vi "phan_dieukhiengoc.vi"() -> ()   [LabVIEW 2019]
uses:
  <vilib>/Platform/TimedLoop/XDataNode/timing_clust.ctl
  <vilib>/Platform/TimedLoop/XDataNode/nitl_modes.ctl
  <vilib>/Platform/TimedLoop/XDataNode/wakeup.ctl
  <vilib>/platform/TimedLoop/XDataNode/XDataNode.xnode
  <vilib>/Platform/TimedLoop/XDataNode/XDNodeRunTimeDep.lvlib
  <vilib>/ptbypt/NI_PtbyPt.lvlib
panel:
  out "wdk":dbl
  out "phi_sp":dbl
  in  "Kiw":dbl
  in  "Kpw":dbl
  in  "Kdw":dbl=2.0
  out "phi_ph":dbl
  out "Vxdk":dbl
  out "Vydk":dbl
  in  "Kdv3":dbl
  in  "Kiv3":dbl=28.5
  in  "Kpv3":dbl=0.7
  in  "Kdv2":dbl
  in  "Kiv2":dbl=28.5
  in  "Kpv2":dbl=0.7
  out "Ts":dbl=10.0
  out "TOA DO 2":dbl[][](array[numeric])
  out "sailechxy":cluster{"e_phi":dbl, "e_x":dbl, "e_y":dbl}(graph)
  in  "Kdxy":dbl
  in  "Kixy":dbl
  in  "Kpxy":dbl=4.0
  in  "?":enum32{"DUONG 2", "DUONGTRON", "NHAP DIEM"}(tab)
  in  "xstart":dbl format="%#_13g"
  in  "xend":dbl=2.0
  in  "time2":dbl=10.0
  in  "R":dbl=0.8
  in  "phi_end":dbl=15.71
  in  "phi_start":dbl=3.14159 format="%#_13g"
  in  "time1":dbl=30.0
  out "output variable":dbl
  in  "y2":dbl
  in  "x1":dbl
  in  "x2":dbl
  in  "time3":dbl=10.0
  in  "x3":dbl
  in  "y3":dbl
  in  "y1":dbl
  in  "x4":dbl
  in  "y4":dbl
  out "V_ph":dbl
  out "w_ph3":dbl
  out "w_ph2":dbl
  out "w_ph1":dbl
  in  "RESETMAP":bool=TRUE caption="Reset"
  out "duty3":dbl
  out "duty2":dbl
  out "duty1":dbl
  in  "RESET":bool
  out "Y_sp":dbl
  out "X_sp":dbl
  out "Y_ph":dbl
  out "X_ph":dbl
  out "Map":cluster{"Y":dbl[], "Y":dbl[]}[](graph)
  out "V3_sp":dbl
  out "V3_ph":dbl
  out "VAN TOC":T1(graph)
  in  "Kdv1":dbl
  in  "Kiv1":dbl=28.5
  in  "Kpv1":dbl=0.7
  out "V2_ph":dbl
  out "V1_ph":dbl
  out "V2_sp":dbl
  out "V1_sp":dbl
  in  "START":bool
  # "HE THONG"
  # "PID VI TRI"
  # "PID TOC DO"
  # "DUTY"
  # "VI TRI DIEU KHIEN\n(m)"
  # "VI TRI PHAN HOI\n(m)"
  # "TOC DO PHAN HOI (rad/s)"
  # "VAN TOC DIEU KHIEN\n(m/s)"
  # "VAN TOC PHAN HOI\n(m/s)"
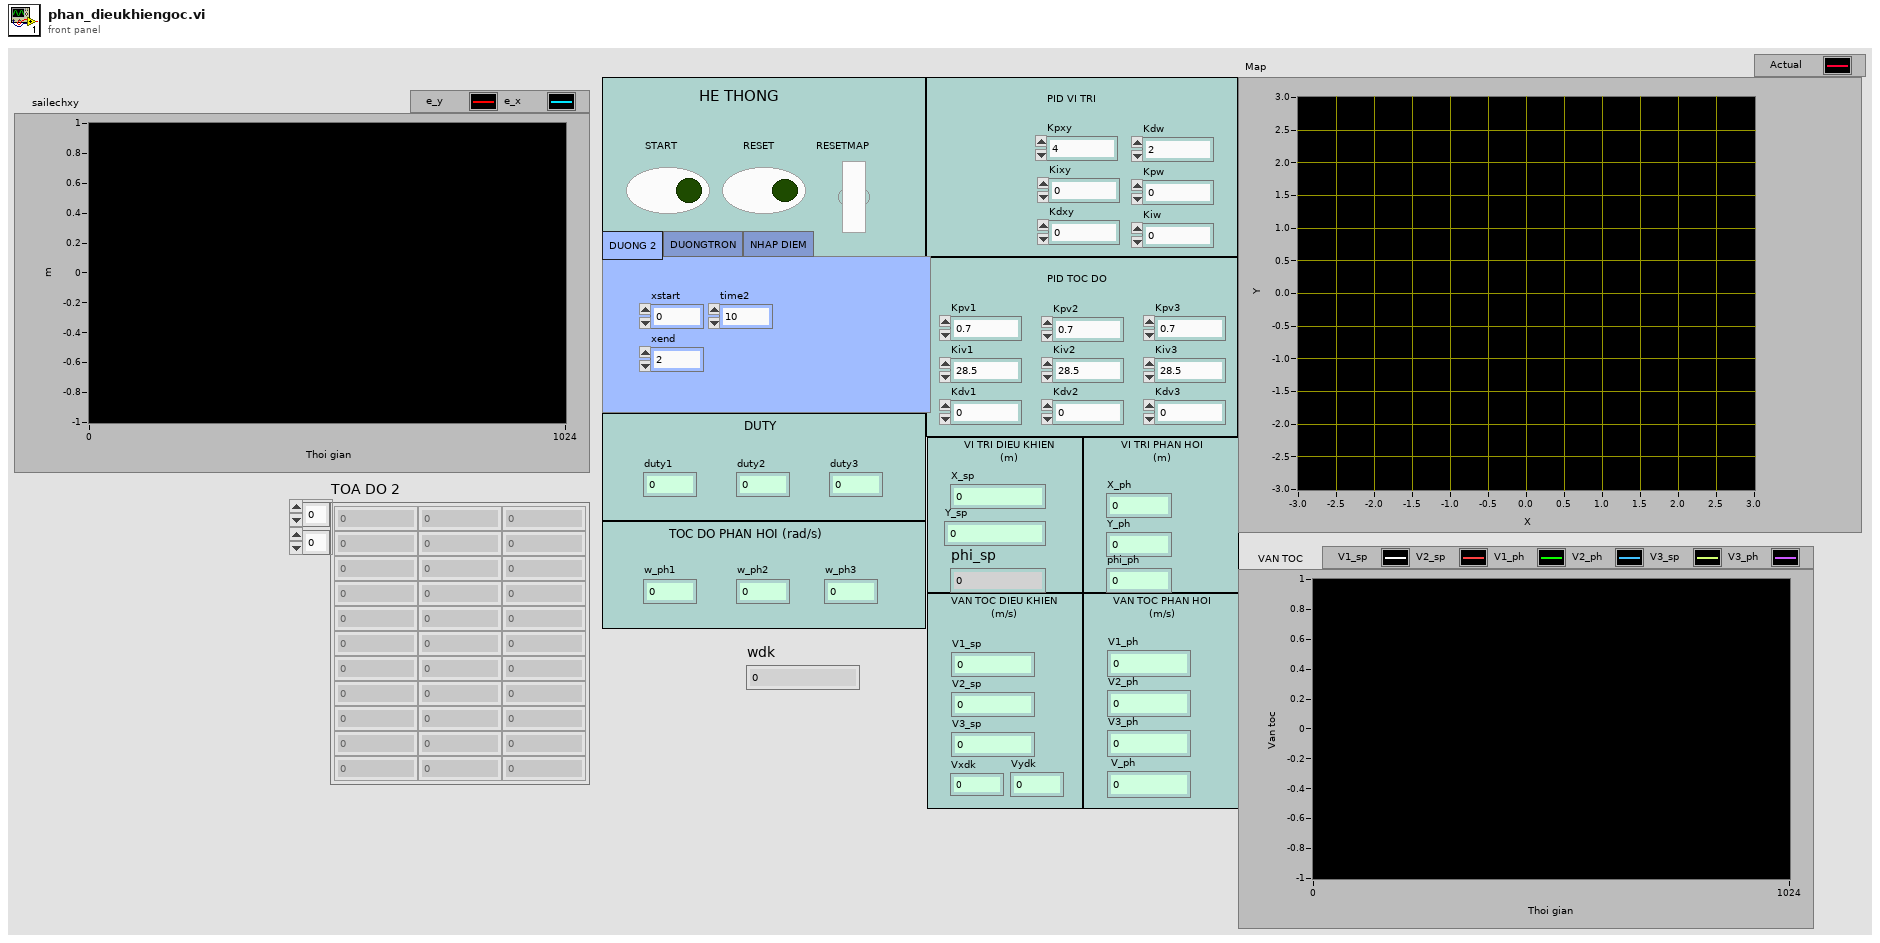
[diagram p1: front panel]
types:
  T1 = cluster{dbl, dbl, "V1_ph":dbl, "V2_ph":dbl, dbl, "V3_ph":dbl}
  T2 = typedef "XDNodeRunTimeDep.lvlib/timing_clust.ctl" = cluster{"Expected End [f-1]":u64, "Actual End [f-1]":u64, "Finished Late? [f-1]":bool, "Expected End [i-1]":u64, "Actual End [i-1]":u64, "Finished Late? [i-1]":bool, "Expected Start [i]":u64, "Actual Start [i]":u64, "Expected Start [f]":u64, "Actual Start [f]":u64, "Source Name":string, "Structure Name":string, "Period":i64, "Deadline":i64, "Offset":i64, "Start":i64, "Priority":i32, "Timeout":i32, "Mode":T3, "Wakeup Reason":T4, "Error":errorcluster, "Source Type":string, "Secondary Source Type":string, "Global End Time":u64, "Global Start Time":u64, "Frame Duration":u64, "Iteration Duration":u64, "Assigned CPU":i32, "I/O Scan Engine Mode":u32}
  T3 = typedef "XDNodeRunTimeDep.lvlib/nitl_modes.ctl" = enum32{"No Change", "Process missed periods, maintain original phase", "Discard missed periods, maintain original phase", "Process missed periods, ignore original phase", "Discard missed periods, ignore original phase"}
  T4 = typedef "XDNodeRunTimeDep.lvlib/wakeup.ctl" = enum32{"Normal", "Aborted", "Asynchronous wakeup", "Timing source error", "Timed loop error", "Timeout"}
  T5 = cluster{"V1_sp":dbl, "V_ph1":dbl, "V2_sp":dbl, "V_ph2":dbl, "V3_sp":dbl, "V_ph3":dbl}
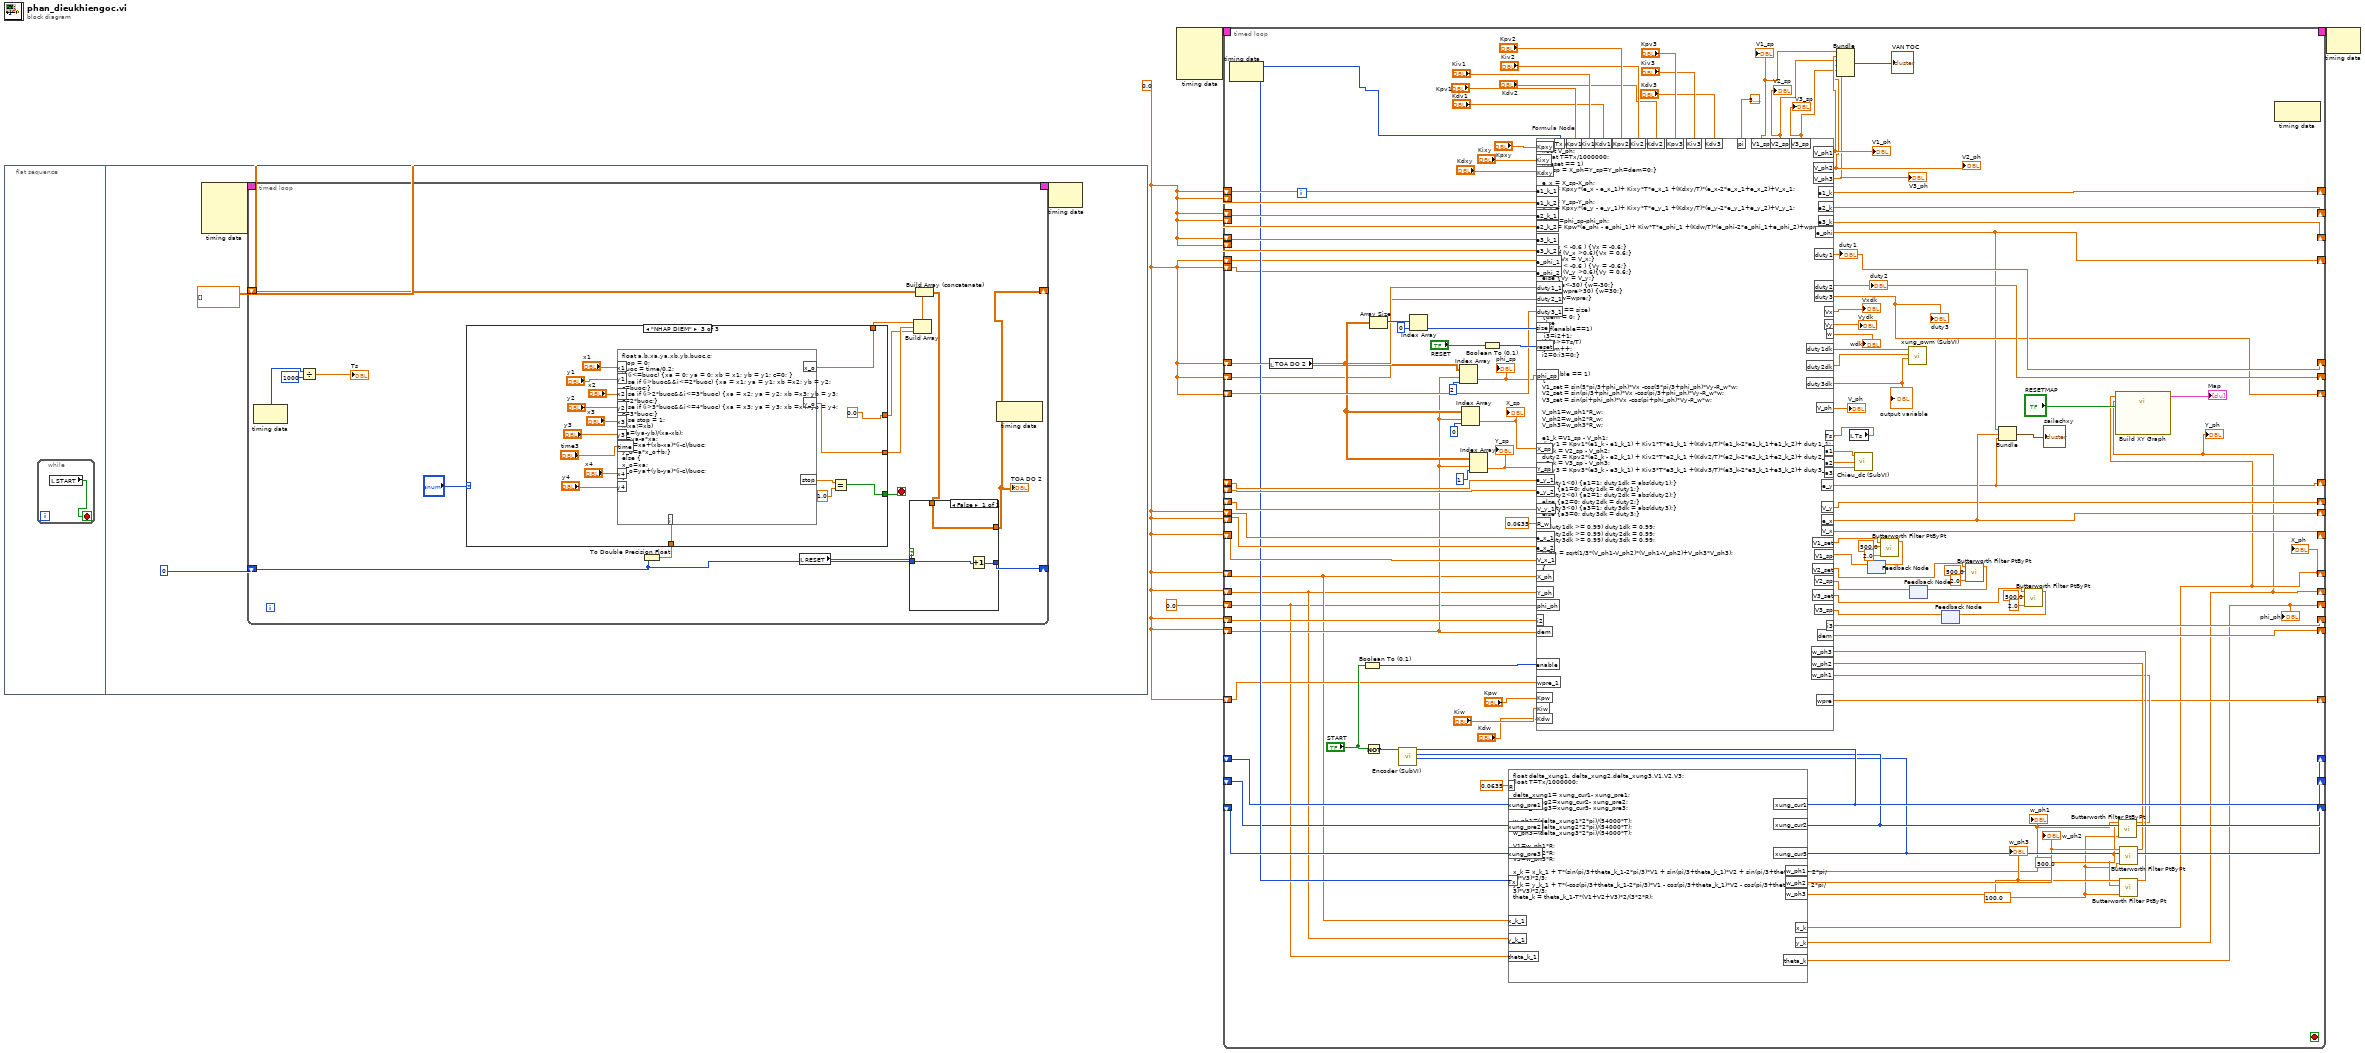
[diagram p0: block diagram]
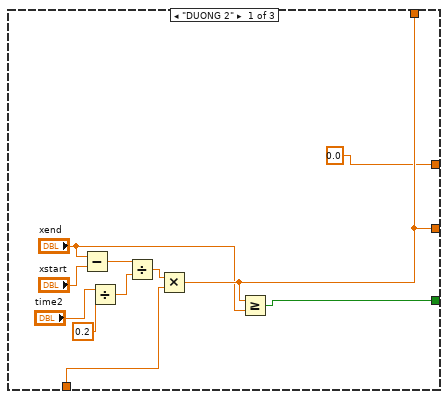
[diagram p2: hidden frame]
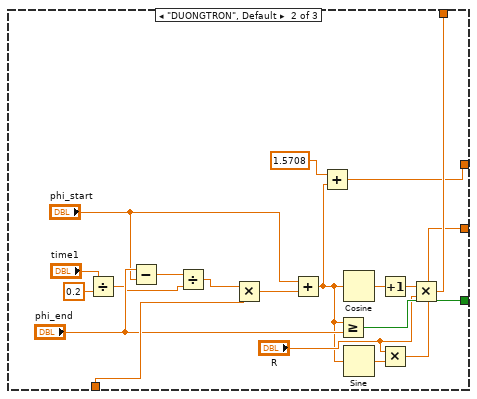
[diagram p3: hidden frame]
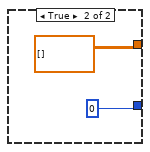
[diagram p4: hidden frame]
diagram:
  w2 = 0.0 ("e1")
  n1 = flat-sequence {
    frame #0 {
      n2 = while {
        stop <- w5 stop-if-true
        n3 = local read "START"() -> (w5:bool)
      }
    }
    frame #1 {
      n4 = node-c288() -> (w9:T2)  [unwired: 4 in]
      n5 = timed-loop {
        timing: w9 -> [_]
        timing-out: [_] -> w8
        shift-right: [w17] -> _
        shift-left: dbl[][] [] -> [w23]
        shift-right: [w21] -> _
        shift-left: 0 -> [w20]
        stop <- w14 stop-if-true
        n6 = node-c288() -> (w16:i64)  [unwired: 1 in]
        n7 = Divide(x=w16, y=i64 1000) -> (x/y=→"Ts":dbl)
        n8 = To Double Precision Float(number=w20) -> (double precision float=w25:dbl)
        n9 = case shown="\"NHAP DIEM\"" "?" {
          tunnel: w25 -> [w33 w55 w71]
          tunnel: [w32 w50 w64] -> w19
          tunnel: [w32 w49 w59] -> w18
          tunnel: [w30 w48 w61] -> w14
          tunnel: [0.0 w37 0.0] -> w10
          frame "DUONG 2" {
            n10 = Subtract(x="xend", y="xstart") -> (x-y=w35:dbl)
            n11 = Divide(x="time2", y=0.2) -> (x/y=w27:dbl)
            n12 = Divide(x=w35, y=w27) -> (x/y=w34:dbl)
            n13 = Multiply(x=w34, y=w33) -> (x*y=w32:dbl)
            n14 = Greater Or Equal?(x=w32, y="xend") -> (x >= y?=w30:bool)
          }
          frame "DUONGTRON", Default {
            n15 = Divide(x="time1", y=0.2) -> (x/y=w41:dbl)
            n16 = Subtract(x="phi_end", y="phi_start") -> (x-y=w45:dbl)
            n17 = Divide(x=w45, y=w41) -> (x/y=w44:dbl)
            n18 = Multiply(x=w44, y=w55) -> (x*y=w54:dbl)
            n19 = Add(x="phi_start", y=w54) -> (x+y=w38:dbl)
            n20 = Add(x=1.5708, y=w38) -> (x+y=w37:dbl)
            n21 = Greater Or Equal?(x=w38, y="phi_end") -> (x >= y?=w48:bool)
            n22 = Cosine(x=w38) -> (cos(x)=w53:dbl)
            n23 = Sine(x=w38) -> (sin(x)=w51:dbl)
            n24 = Increment(x=w53) -> (x+1=w52:dbl)
            n25 = Multiply(x="R", y=w51) -> (x*y=w49:dbl)
            n26 = Multiply(x=w52, y="R") -> (x*y=w50:dbl)
          }
          frame "NHAP DIEM" {
            n27 = formula code="float a,b,xa,ya,xb,yb,buoc,c;\nstop = 0;\nbuoc = time/0.2;\nif (i<=buoc) {xa = 0; ya = 0; xb = x1; yb = y1; c=0; }\nelse if (i>buoc&&i<=2*buoc) {xa = x1; ya = y1; xb =x2; yb = y2; c=buoc;}\nelse if (i>2*buoc&&i<=3*buoc) {xa = x2; ya = y2; xb =x3; yb = y3; c=2*buoc;}\nelse if (i>3*buoc&&i<=4*buoc) {xa = x3; ya = y3; xb =x4; yb = y4; c=3*buoc;}\nelse stop = 1;\nif(xa!=xb)\n{a=(ya-yb)/(xa-xb);\nb=ya-a*xa;\nx_o=xa+(xb-xa)*(i-c)/buoc;\ny_o=a*x_o+b;}\nelse {\nx_o=xa;\ny_o=ya+(yb-ya)*(i-c)/buoc;\n}"("i"=w71, "x1"="x1", "y1"="y1", "x2"="x2", "y2"="y2", "x3"="x3", "y3"="y3", "time"="time3", "x4"="x4", "y4"="y4") -> ("x_o"=w64:dbl, "y_o"=w59:dbl, "stop"=w63:dbl)
            n28 = Equal?(x=w63, y=1.0) -> (x = y?=w61:bool)
          }
        }
        n29 = local read "RESET"() -> (w13:bool)
        n30 = Build Array(w19, w18, w10) -> (w24:dbl[])
        n31 = Build Array (concatenate)(w23, w24) -> (w22:dbl[][])
        n32 = case shown="False" w13 {
          tunnel: w22 -> [w74 _]
          tunnel: [w74 dbl[][] []] -> w17
          tunnel: [w73 0] -> w21
          tunnel: w20 -> [w72 _]
          frame False {
            n33 = Increment(x=w72) -> (x+1=w73:i32)
          }
          frame True {
          }
        }
        "TOA DO 2" <- w17
        n34 = node-c288() -> ()  [unwired: 1 in, 1 out]
      }
      n35 = node-c288(w8) -> ()  [unwired: 1 out]
    }
  }
  n36 = node-c288() -> (w4:T2)  [unwired: 4 in]
  n37 = timed-loop {
    timing: w4 -> [_]
    timing-out: [_] -> w3
    shift-right: [w205] -> _
    shift-left: w2 -> [w203]
    shift-right: [w204] -> _
    shift-left: w2 -> [w162]
    shift-right: [w196] -> _
    shift-left: w2 -> [w195]
    shift-right: [w90] -> _
    shift-left: w2 -> [w87]
    shift-right: [w89] -> _
    shift-left: w2 -> [w86]
    shift-right: [w194] -> _
    shift-left: w2 -> [w102]
    shift-right: [w174] -> _
    shift-left: w2 -> [w175]
    shift-right: [w173] -> _
    shift-left: w2 -> [w171]
    shift-right: [w172] -> _
    shift-left: w2 -> [w99]
    shift-right: [w100] -> _
    shift-left: w2 -> [w170]
    shift-right: [w165] -> _
    shift-left: _ -> [w167]
    shift-right: [w164] -> _
    shift-left: _ -> [w96]
    shift-right: [w163] -> _
    shift-left: _ -> [w166]
    shift-right: [w115] -> _
    shift-left: w2 -> [w157]
    shift-right: [w155] -> _
    shift-left: w2 -> [w156]
    shift-left: w2 -> [w151]
    shift-left: w2 -> [w150]
    shift-left: w2 -> [w149]
    shift-left: w2 -> [w148]
    shift-right: [w106] -> _
    shift-left: _ -> [w111]
    shift-right: [w113] -> _
    shift-left: _ -> [w112]
    shift-left: _ -> [w110]
    shift-right: [w88] -> _
    shift-left: 0.0 ("phi_ph") -> [w85]
    shift-right: [w82] -> _
    shift-left: w2 -> [w98]
    shift-left: w2 -> [w97]
    shift-right: [w94] -> _
    shift-left: w2 -> [w95]
    stop <- _ stop-if-true
    w142 = 100.0 ("flw")
    w143 = 500.0 ("sampling freq: fs")
    n38 = node-c288() -> (w105:i64)  [unwired: 1 in]
    n39 = local read "TOA DO 2"() -> (w103:dbl[][])
    n40 = Boolean To (0,1)(Boolean="START") -> (0, 1=w202:i16)
    n41 = Not(x="START") -> (.not. x?=w177:bool)
    n42 = Array Size(array=w103) -> (size(s)=w190:i32[])
    n43 = call "Encoder (SubVI).vi"("Boolean"=w177) -> ("Counter Value3"=w163:i32, "Counter Value 2"=w164:i32, "Counter Value"=w165:i32)  [unwired: 8 in]
    n44 = Index Array(array=w190, index=0) -> (element=w188:i32)
    n45 = Index Array(array=w103, index (row)=w102, index (col)=2 ("disabled index (col)")) -> (element=w101:dbl)
    "phi_sp" <- w101
    n46 = Index Array(array=w103, index (row)=w102, index (col)=0 ("disabled index (col)")) -> (element=w192:dbl)
    "X_sp" <- w192
    n47 = Index Array(array=w103, index (row)=w102, index (col)=1 ("disabled index (col)")) -> (element=w191:dbl)
    "Y_sp" <- w191
    n48 = Boolean To (0,1)(Boolean="RESET") -> (0, 1=w187:i16)
    n49 = formula code="float delta_xung1, delta_xung2,delta_xung3,V1,V2,V3;\nfloat T=Tx/1000000;\n\ndelta_xung1= xung_cur1- xung_pre1;\ndelta_xung2=xung_cur2- xung_pre2;\ndelta_xung3=xung_cur3- xung_pre3; \n\nw_ph1=(delta_xung1*2*pi)/(54000*T);\nw_ph2=(delta_xung2*2*pi)/(54000*T);\nw_ph3=(delta_xung3*2*pi)/(54000*T);\n\nV1=w_ph1*R;\nV2=w_ph2*R;\nV3=w_ph3*R;\n\nx_k = x_k_1 + T*(sin(pi/3+theta_k_1-2*pi/3)*V1 + sin(pi/3+theta_k_1)*V2 + sin(pi/3+theta_k_1 + 2*pi/3)*V3)*2/3;\ny_k = y_k_1 + T*(-cos(pi/3+theta_k_1-2*pi/3)*V1 - cos(pi/3+theta_k_1)*V2 - cos(pi/3+theta_k_1 + 2*pi/3)*V3)*2/3;\ntheta_k = theta_k_1-T*(V1+V2+V3)*2/(3*2*R);"("xung_pre1"=w167, "xung_pre2"=w96, "xung_pre3"=w166, "xung_cur1"=w165, "xung_cur2"=w164, "xung_cur3"=w163, "Tx"=w105, "x_k_1"=w87, "y_k_1"=w86, "theta_k_1"=w85, "R"=0.0635 ("input variable")) -> ("w_ph1"=w133:dbl, "w_ph2"=w145:dbl, "w_ph3"=w144:dbl, "x_k"=w90:dbl, "y_k"=w89:dbl, "theta_k"=w88:dbl)
    "X_ph" <- w90
    "Y_ph" <- w89
    "w_ph1" <- w133
    "w_ph2" <- w145
    "w_ph3" <- w144
    "phi_ph" <- w88
    n50 = local read "Ts"() -> (w107:dbl)
    n51 = feedback #1() -> (w123:dbl)  [unwired: 1 in]
    n52 = feedback #2() -> (w120:dbl)  [unwired: 1 in]
    n53 = feedback #3() -> (w117:dbl)  [unwired: 1 in]
    n54 = call "Build XY Graph"("Reset"="RESETMAP", "Y Input"=w89, "X Input"=w90) -> ("XY Graph"=→"Map":cluster{"X":dbl[], "Y":dbl[]}[])  [unwired: 7 in, 1 out]
    n55 = call <vilib>:"Butterworth Filter PtByPt.vi"("low cutoff freq: fl"=w142, "sampling freq: fs"=w143, "x"=w133) -> ("Filtered x"=w132:dbl)  [unwired: 6 in, 1 out]
    n56 = call <vilib>:"Butterworth Filter PtByPt.vi"("low cutoff freq: fl"=w142, "sampling freq: fs"=w143, "x"=w145) -> ("Filtered x"=w141:dbl)  [unwired: 6 in, 1 out]
    n57 = call <vilib>:"Butterworth Filter PtByPt.vi"("low cutoff freq: fl"=w142, "sampling freq: fs"=w143, "x"=w144) -> ("Filtered x"=w140:dbl)  [unwired: 6 in, 1 out]
    n58 = formula code="float V,Vtest, S_sp, S_ph, Vx, Vy,w;\nfloat V_ph;\n float T=Tx/1000000;\nif(reset == 1)\n{X_sp = X_ph=Y_sp=Y_ph=dem=0;}\n\ne_x = X_sp-X_ph; \nV_x = Kpxy*(e_x - e_x_1)+ Kixy*T*e_x_1 +(Kdxy/T)*(e_x-2*e_x_1+e_x_2)+V_x_1;\n\ne_y = Y_sp-Y_ph; \nV_y = Kpxy*(e_y - e_y_1)+ Kixy*T*e_y_1 +(Kdxy/T)*(e_y-2*e_y_1+e_y_2)+V_y_1;\n\ne_phi=phi_sp-phi_ph;\nwpre= Kpw*(e_phi - e_phi_1)+ Kiw*T*e_phi_1 +(Kdw/T)*(e_phi-2*e_phi_1+e_phi_2)+wpre_1;\n\n\nif (V_x < -0.6 ) {Vx = -0.6;} \nelse if (V_x >0.6){Vx = 0.6;}\nelse {Vx = V_x;}\nif (V_y < -0.6 ) {Vy = -0.6;} \nelse if (V_y >0.6){Vy = 0.6;}\nelse {Vy = V_y;}\nif (wpre<-30) {w=-30;}\nelse if(wpre>30) {w=30;}\nelse {w=wpre;}\n\nif(dem == size)\n{dem = 0; }\nelse\n{ if(enable==1)\n i3=i2+1;\nif (i3>=Ts/T)\n{dem++;\ni2=0;i3=0;}\n\n\nif(enable == 1)\n{\nV1_set = sin(5*pi/3+phi_ph)*Vx -cos(5*pi/3+phi_ph)*Vy-R_w*w;\nV2_set = sin(pi/3+phi_ph)*Vx -cos(pi/3+phi_ph)*Vy-R_w*w;\nV3_set = sin(pi+phi_ph)*Vx -cos(pi+phi_ph)*Vy-R_w*w;\n\nV_ph1=w_ph1*R_w;\nV_ph2=w_ph2*R_w;\nV_ph3=w_ph3*R_w;\n\ne1_k =V1_sp - V_ph1;\nduty1 = Kpv1*(e1_k - e1_k_1) + Kiv1*T*e1_k_1 +(Kdv1/T)*(e1_k-2*e1_k_1+e1_k_2)+ duty1_1;\ne2_k = V2_sp - V_ph2;\nduty2 = Kpv2*(e2_k - e2_k_1) + Kiv2*T*e2_k_1 +(Kdv2/T)*(e2_k-2*e2_k_1+e2_k_2)+ duty2_1;\ne3_k = V3_sp - V_ph3;\nduty3 = Kpv3*(e3_k - e3_k_1) + Kiv3*T*e3_k_1 +(Kdv3/T)*(e3_k-2*e3_k_1+e3_k_2)+ duty3_1;\n\nif(duty1<0) {a1=1; duty1dk = abs(duty1);}\nelse {a1=0; duty1dk = duty1;}\nif(duty2<0) {a2=1; duty2dk = abs(duty2);}\nelse {a2=0; duty2dk = duty2;}\nif(duty3<0) {a3=1; duty3dk = abs(duty3);}\nelse {a3=0; duty3dk = duty3;}\n\nif(duty1dk >= 0.99) duty1dk = 0.99;\nif(duty2dk >= 0.99) duty2dk = 0.99;\nif(duty3dk >= 0.99) duty3dk = 0.99;\n\nV_ph = sqrt(1/3*(V_ph1-V_ph2)*(V_ph1-V_ph2)+V_ph3*V_ph3);\n\n}\n}"("Kpv1"="Kpv1", "Kiv1"="Kiv1", "Kdv1"="Kdv1", "pi"=3.141592653589793, "e1_k_1"=w203, "e2_k_1"=w162, "enable"=w202, "Tx"=w105, "e3_k_1"=w195, "X_ph"=w87, "X_sp"=w192, "Y_sp"=w191, "Y_ph"=w86, "dem"=w102, "size"=w188, "reset"=w187, "i2"=w175, "duty1_1"=w171, "duty2_1"=w99, "duty3_1"=w170, "w_ph1"=w132, "w_ph2"=w141, "w_ph3"=w140, "e_x_1"=w157, "V_x_1"=w156, "Kpxy"="Kpxy", "Kixy"="Kixy", "Kdxy"="Kdxy", "e1_k_2"=w151, "e2_k_2"=w150, "e3_k_2"=w149, "e_x_2"=w148, "Ts"=w107, "Kpv2"="Kpv2", "Kiv2"="Kiv2", "Kdv2"="Kdv2", "Kpv3"="Kpv3", "Kiv3"="Kiv3", "Kdv3"="Kdv3", "V1_sp"=w123, "V2_sp"=w120, "V3_sp"=w117, "R_w"=0.0635 ("input variable"), "e_y_1"=w111, "e_y_2"=w110, "V_y_1"=w112, "phi_sp"=w101, "phi_ph"=w85, "e_phi_1"=w98, "e_phi_2"=w97, "wpre_1"=w95, "Kpw"="Kpw", "Kiw"="Kiw", "Kdw"="Kdw") -> ("V1_sp"=w185:dbl, "V_ph1"=w184:dbl, "V_ph2"=w182:dbl, "e1_k"=w205:dbl, "e2_k"=w204:dbl, "V2_sp"=w183:dbl, "duty1"=w173:dbl, "duty2"=w172:dbl, "e3_k"=w196:dbl, "V_ph3"=w181:dbl, "V3_sp"=w180:dbl, "duty3"=w100:dbl, "a1"=w176:dbl, "a2"=w169:dbl, "a3"=w168:dbl, "dem"=w194:dbl, "i3"=w174:dbl, "duty1dk"=w161:dbl, "duty2dk"=w160:dbl, "duty3dk"=w159:dbl, "V_ph"=→"V_ph":dbl, "e_x"=w115:dbl, "V_x"=w155:dbl, "V1_set"=w125:dbl, "V2_set"=w122:dbl, "V3_set"=w119:dbl, "e_y"=w106:dbl, "V_y"=w113:dbl, "Vx"=→"Vxdk":dbl, "Vy"=→"Vydk":dbl, "e_phi"=w82:dbl, "wpre"=w94:dbl, "w"=→"wdk":dbl)
    "V1_sp" <- w185
    "V2_sp" <- w183
    "V1_ph" <- w184
    "V2_ph" <- w182
    "V3_ph" <- w181
    "V3_sp" <- w180
    "duty1" <- w173
    "duty2" <- w172
    "duty3" <- w100
    "output variable" <- w159
    n59 = Bundle("V1_sp"=w185, "V_ph1"=w184, "V2_sp"=w183, "V_ph2"=w182, "V3_sp"=w180, "V_ph3"=w181) -> (→"VAN TOC":T5)  [unwired: 1 in]
    n60 = call "Chieu_dc (SubVI).vi"("a3"=w168, "a2"=w169, "a1"=w176) -> ()
    n61 = call <vilib>:"Butterworth Filter PtByPt.vi"("low cutoff freq: fl"=2.0, "sampling freq: fs"=500.0, "x"=w125) -> ("Filtered x"=w124:dbl)  [unwired: 6 in, 1 out]
    n62 = feedback-in #1(w124) -> ()
    n63 = call "xung_pwm (SubVI).vi"("duty3 in"=w159, "duty2 in"=w160, "duty1 in"=w161) -> ()  [unwired: 6 in, 3 out]
    n64 = call <vilib>:"Butterworth Filter PtByPt.vi"("low cutoff freq: fl"=2.0, "sampling freq: fs"=500.0, "x"=w122) -> ("Filtered x"=w121:dbl)  [unwired: 6 in, 1 out]
    n65 = feedback-in #2(w121) -> ()
    n66 = Bundle("e_phi"=w82, "e_x"=w115, "e_y"=w106) -> (→"sailechxy":cluster{"e_phi":dbl, "e_x":dbl, "e_y":dbl})  [unwired: 1 in]
    n67 = call <vilib>:"Butterworth Filter PtByPt.vi"("low cutoff freq: fl"=2.0, "sampling freq: fs"=500.0, "x"=w119) -> ("Filtered x"=w118:dbl)  [unwired: 6 in, 1 out]
    n68 = feedback-in #3(w118) -> ()
    n69 = node-c288() -> ()  [unwired: 1 in, 1 out]
  }
  n70 = node-c288(w3) -> ()  [unwired: 1 out]
